vi "generate-analog-out-waveform.vi"(0 "EMG Data File":path=path "C:/data/analog-out-svm.csv", 1 "physical Output channels":tag="DAQ1/ao0", 2 "Delta T":dbl=0.0005, 5 "error in":errorcluster) -> (14 "Waveform Graph":waveform(dbl)(graph) caption="Output Waveform", 19 "error out":errorcluster)   [LabVIEW 2020]
uses:
  <vilib>/Utility/error.llb/DialogType.ctl
  <vilib>/DAQmx/write.llb/DAQmx Write (Analog 1D DBL 1Chan NSamp).vi
  <vilib>/Utility/file.llb/Read From Spreadsheet File (DBL).vi
  <vilib>/DAQmx/create/channels.llb/DAQmx Create Channel (AO-Voltage-Basic).vi
  <vilib>/DAQmx/configure/timing.llb/DAQmx Timing (Use Waveform).vi
  <vilib>/DAQmx/miscellaneous.llb/DAQmx Fill In Error Info.vi
panel:
  in  "Column":i32
  in  "Minimum Value":dbl=-10.0 format="%0.2f"
  in  "Maximum Value":dbl=10.0 format="%0.2f"
  in  "stop":bool
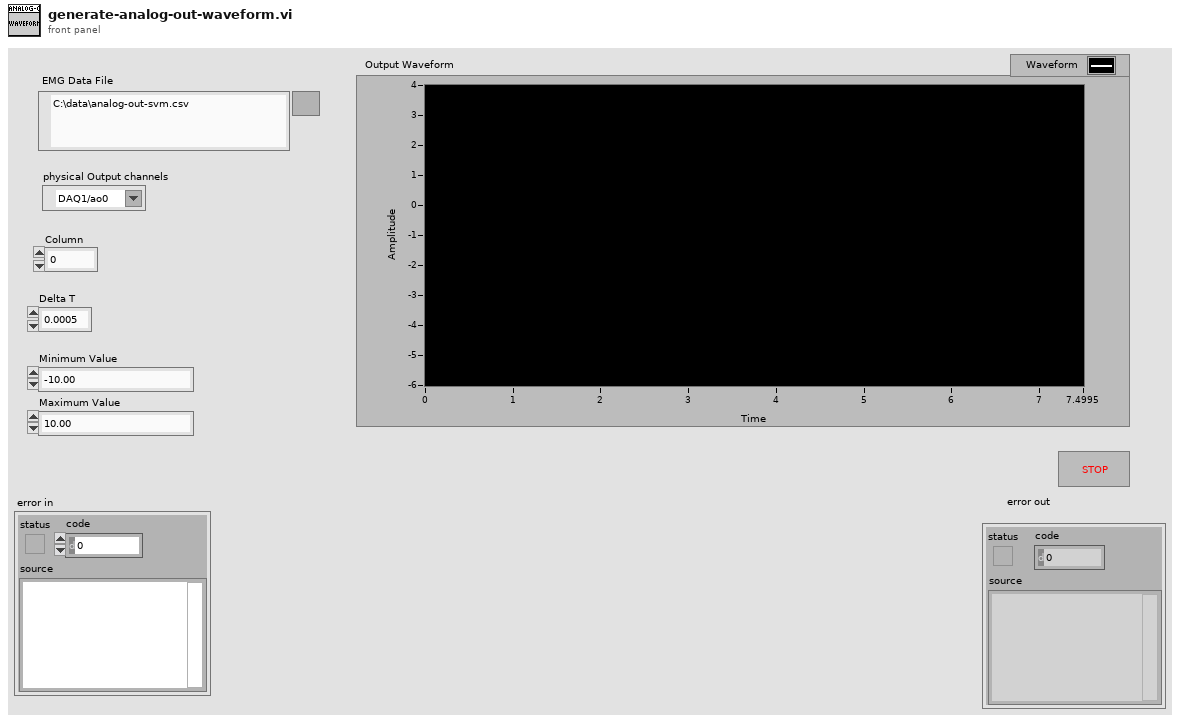
[diagram p1: front panel]
types:
  T1 = typedef "DialogType.ctl" = u16
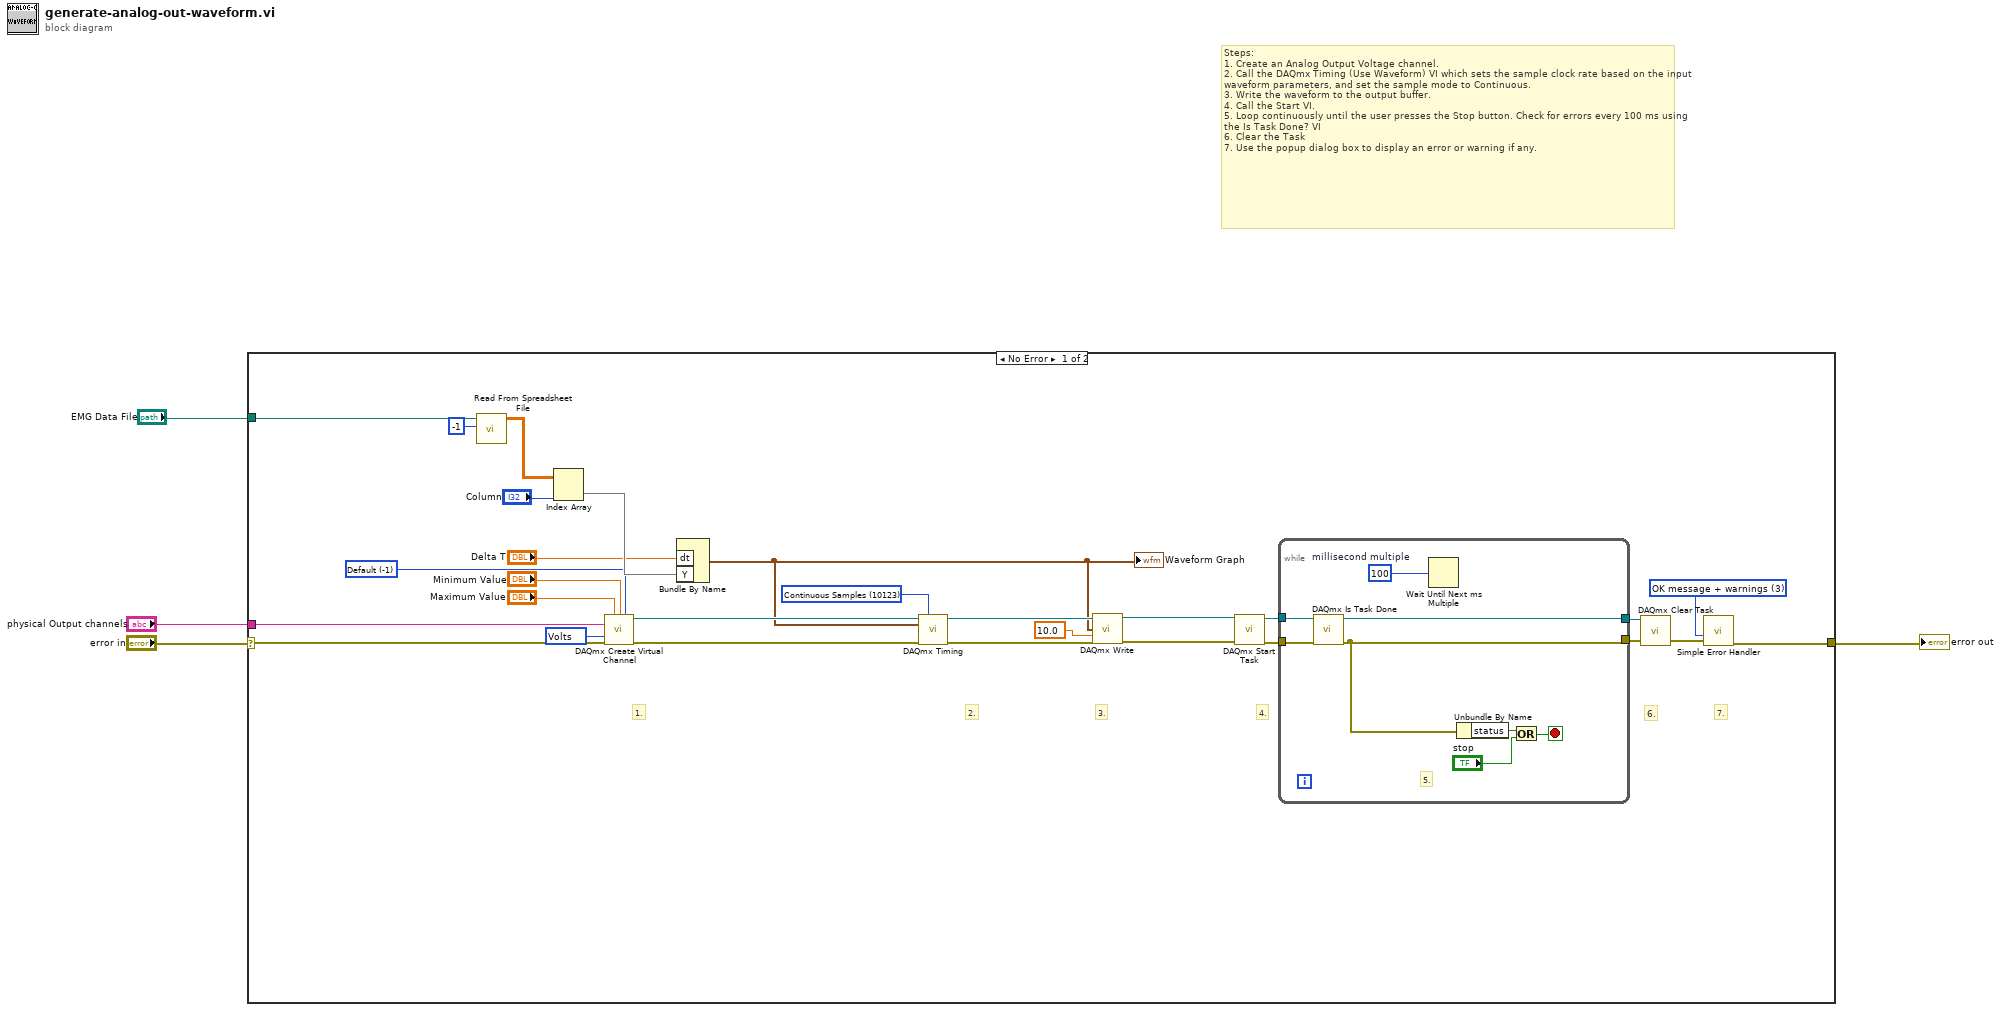
[diagram p0: block diagram]
diagram:
  # "Steps: \n1. Create an Analog Output Voltage channel.\n2. Call the DAQmx Timing (Use Waveform) VI which sets the sample clock rate based on the input waveform parameters, and set the sample mode to Continuous.\n3. Write the waveform to the output buffer.\n4. Call the Start VI.\n5. Loop continuously until the user presses the Stop button. Check for errors every 100 ms using the Is Task Done? VI\n6. Clear the Task\n7. Use the popup dialog box to display an error or warning if any."
  n1 = case shown="No Error" "error in" {
    selector: "error in" -> [w7 w41]
    tunnel: [w11 w41] -> w4
    tunnel: "physical Output channels" -> [w6 _]
    tunnel: "EMG Data File" -> [w5 _]
    frame No Error {
      w9 = 10348 items=["Volts"=10348, "From Custom Scale"=10065] ("units")
      w10 = -1 items=["Default"=-1, "RSE"=10083, "Differential"=10106, "Pseudodifferential"=12529] ("output terminal configuration")
      w21 = T1 3 items=["no dialog", "OK message", "continue or stop message", "OK message + warnings", "continue/stop + warnings"] ("type of dialog (OK msg:1)")
      w31 = 10123 items=["Finite Samples"=10178, "Continuous Samples"=10123] ("sample mode")
      # "7."
      # "6."
      # "4."
      # "3."
      # "2."
      # "1."
      n2 = call-poly <vilib>:"Read From Spreadsheet File.vi"("number of rows (all:-1)"=-1, "file path (dialog if empty)"=w5) -> ("all rows"=w16:dbl[][])  [unwired: 5 in, 4 out]
      n3 = Index Array(array=w16, index (col)="Column") -> (element=w17:dbl[])  [unwired: 1 in]
      n4 = call-poly <vilib>:"DAQmx Create Virtual Channel.vi"("maximum value"="Maximum Value", "minimum value"="Minimum Value", "output terminal configuration"=w10, "physical channels"=w6, "units"=w9, "error in"=w7) -> ("task out"=w12:refnum<k21>, "error out"=w13:errorcluster)  [unwired: 8 in]
      n5 = Bundle By Name("dt"="Delta T", "Y"=w17) -> (w8:waveform(dbl))  [unwired: 1 in]
      "Waveform Graph" <- w8
      n6 = call-poly <vilib>:"DAQmx Timing.vi"("task/channels in"=w12, "sample mode"=w31, "waveform"=w8, "error in"=w13) -> ("task out"=w24:refnum<k21>, "error out"=w23:errorcluster)  [unwired: 10 in]
      n7 = call-poly <vilib>:"DAQmx Write.vi"("task/channels in"=w24, "data"=w8, "timeout"=10.0 ("Wirite Timeout"), "error in"=w23) -> ("task out"=w28:refnum<k21>, "error out"=w27:errorcluster)  [unwired: 9 in, 1 out]
      n8 = call <vilib>:"DAQmx Start Task.vi"("task/channels in"=w28, "error in"=w27) -> ("task out"=w22:refnum<k21>, "error out"=w25:errorcluster)  [unwired: 12 in]
      n9 = while {
        tunnel: w22 -> [w40]
        tunnel: [w39] -> w20
        tunnel: w25 -> [w38]
        tunnel: [w37] -> w19
        stop <- w35 stop-if-true
        w36 = u32 100  # millisecond multiple
        # "5."
        n10 = call <vilib>:"DAQmx Is Task Done.vi"("task/channels in"=w40, "error in"=w38) -> ("task out"=w39:refnum<k21>, "error out"=w37:errorcluster)  [unwired: 11 in, 1 out]
        n11 = Wait Until Next ms Multiple(millisecond multiple=w36) -> ()  [unwired: 1 out]
        n12 = Unbundle By Name(w37) -> ("status"=w34:bool)
        n13 = Or(x=w34, y="stop") -> (x .or. y?=w35:bool)
      }
      n14 = call <vilib>:"DAQmx Clear Task.vi"("task in"=w20, "error in"=w19) -> ("error out"=w32:errorcluster)  [unwired: 13 in]
      n15 = call <vilib>:"Simple Error Handler.vi"("type of dialog (OK msg:1)"=w21, "error in (no error)"=w32) -> ("error out"=w11:errorcluster)  [unwired: 3 in, 4 out]
    }
    frame Error {
    }
  }
  "error out" <- w4
